vi "MapColor_array2Slide.vi"(6 "SlideValue\nIN":cluster{i32, i32, i32, i32, i32, i32, i32}(slide) scale=1.0..127.0, 7 "numSliders\n(optional)":i32=3, 8 "colormap":u32[](array[numeric])=[0, 196608, 393216, 589824, 786432, 983040, 1179648, 1376256, 1572864, 1769472, 1966080, 2162688, 2359296, 2555904, 2752512, 2949120, 3145728, 3342336, 3538944, 3735552, 3932160, 4128768, 4325376, 4521984, 4718592, 4915200, 5111808, 5308416, 5505024, 5701632, 5898240, 6094848, 6291456, 6488064, 6684672, 6881280, 7077888, 7274496, 7471104, 7667712, 7864320, 8060928, 8257536, 8454144, 8650752, 8847360, 9043968, 9240576, 9437184, 9633792, 9830400, 10027008, 10223616, 10420224, 10616832, 10813440, 11010048, 11206656, 11403264, 11599872, 11796480, 11993088, 12189696, 12386304, 12582912, 12779520, 12976128, 13172736, 13369344, 13565952, 13762560, 13959168, 14155776, 14352384, 14548992, 14745600, 14942208, 15138816, 15335424, 15532032, 15728640, 15925248, 16121856, 16318464, 16515072, 16711680, 16712448, 16713216, 16713984, 16714752, 16715520, 16716288, 16717056, 16717824, 16718592, 16719360, 16720128, 16720896, 16721664, 16722432, 16723200, 16723968, 16724736, 16725504, 16726272, 16727040, 16727808, 16728576, 16729344, 16730112, 16730880, 16731648, 16732416, 16733184, 16733952, 16734720, 16735488, 16736256, 16737024, 16737792, 16738560, 16739328, 16740096, 16740864, 16741632, 16742400, 16743168, 16743936, 16744704, 16745472, 16746240, 16747008, 16747776, 16748544, 16749312, 16750080, 16750848, 16751616, 16752384, 16753152, 16753920, 16754688, 16755456, 16756224, 16756992, 16757760, 16758528, 16759296, 16760064, 16760832, 16761600, 16762368, 16763136, 16763904, 16764672, 16765440, 16766208, 16766976, 16767744, 16768512, 16769280, 16770048, 16770816, 16771584, 16772352, 16773120, 16773888, 16774656, 16775424, 16776192, 16776960, 16776963, 16776966, 16776969, 16776972, 16776975, 16776977, 16776980, 16776983, 16776986, 16776989, 16776992, 16776995, 16776998, 16777001, 16777004, 16777007, 16777009, 16777012, 16777015, 16777018, 16777021, 16777024, 16777027, 16777030, 16777033, 16777036, 16777038, 16777041, 16777044, 16777047, 16777050, 16777053, 16777056, 16777059, 16777062, 16777065, 16777068, 16777070, 16777073, 16777076, 16777079, 16777082, 16777085, 16777088, 16777091, 16777094, 16777097, 16777100, 16777102, 16777105, 16777108, 16777111, 16777114, 16777117, 16777120, 16777123, 16777126, 16777129, 16777132, 16777134, 16777137, 16777140, 16777143, 16777146, 16777149, 16777152, 16777155, 16777158, 16777161, 16777163, 16777166, 16777169, 16777172, 16777175, 16777178, 16777181, 16777184, 16777187, 16777190, 16777193, 16777195, 16777198, 16777201, 16777204, 16777207]) -> (0 "SlideValue\nOUT":cluster{i32, i32, i32, i32, i32, i32, i32}(slide) scale=1.0..127.0, 1 "ActiveColors":i32[](array[numeric]), 2 "ColorFine":u32(colorbox)=16711680, 3 "ColorArray":u32[](array[colorbox]), 4 "ColorRamp":u32[](array[colorbox])=[180, 263349, 526518, 789687, 1052856, 1316026, 1579195, 1842364, 2105533, 2368702, 2631871, 2895040, 3158209, 3421378, 3684548, 3947717, 4145094, 4408263, 4671432, 4934601, 5197770, 5460939, 5724108, 5987278, 6250447, 6513616, 6776785, 7039954, 7303123, 7566292, 7829461, 8092630, 8355800, 8618969, 8882138, 9145307, 9408476, 9671645, 9934814, 10197983, 10461152, 10724322, 10987491, 11250660, 11513829, 11776998, 12040167, 12303336, 12500713, 12763882, 13027052, 13290221, 13553390, 13816559, 14079728, 14342897, 14606066, 14869235, 15132404, 15395574, 15658743, 15921912, 16185081, 16448250, 16448250, 16447222, 16446194, 16445166, 16444138, 16443110, 16442082, 16506590, 16505562, 16504534, 16503506, 16502478, 16501450, 16500422, 16499394, 16498366, 16497595, 16496567, 16495539, 16560047, 16559019, 16557991, 16556963, 16555935, 16554907, 16553879, 16552851, 16551823, 16550795, 16549767, 16548739, 16547711, 16612219, 16611191, 16610163, 16609135, 16608107, 16607079, 16606051, 16605023, 16603995, 16602967, 16601939, 16600911, 16599883, 16664391, 16663363, 16662335, 16661564, 16660536, 16659508, 16658480, 16657452, 16656424, 16655396, 16654368, 16653340, 16717848, 16716820, 16715792, 16714764, 16713736, 16712708, 16711680] caption="Color Ramp", 5 "ColorInizio":u32(colorbox)=180)   [LabVIEW 2010]
panel:
  out "array":i32[](array[numeric])
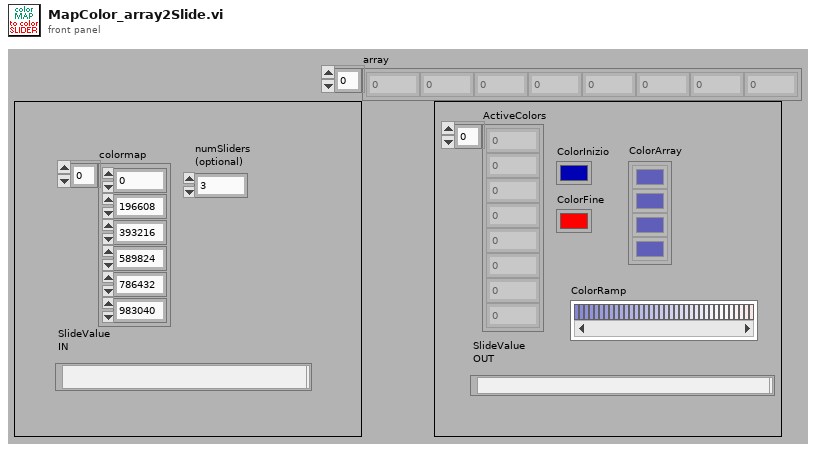
[diagram p1: front panel]
types:
  T1 = cluster{"SlideValue\nIN[0]":i32, "SlideValue\nIN[1]":i32, "SlideValue\nIN[2]":i32, "SlideValue\nIN[3]":i32, "SlideValue\nIN[4]":i32, "SlideValue\nIN[5]":i32, "SlideValue\nIN[6]":i32}
  T2 = cluster{"[0]":i32, "[1]":i32, "[2]":i32, "[3]":i32, "[4]":i32, "[5]":i32, "[6]":i32}
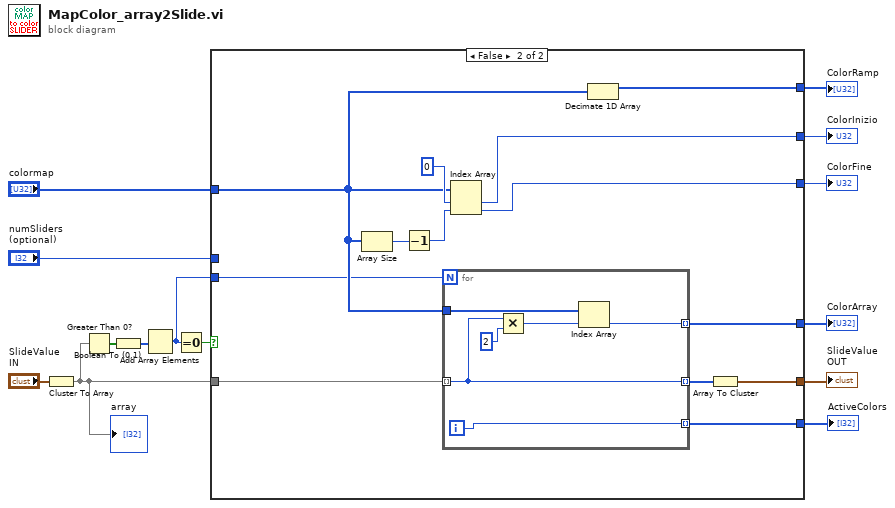
[diagram p0: block diagram]
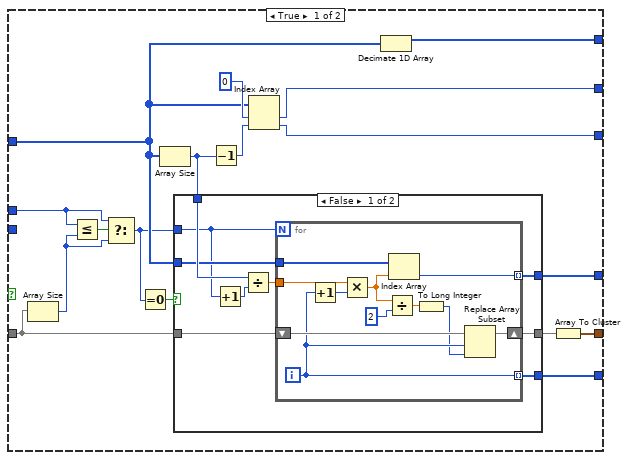
[diagram p2: hidden frame]
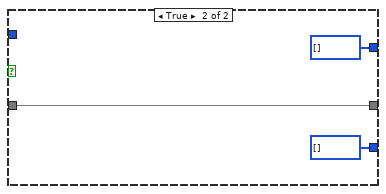
[diagram p3: hidden frame]
diagram:
  n1 = Cluster To Array(cluster="SlideValue\nIN") -> (array=w5:i32[])
  "array" <- w5
  n2 = Greater Than 0?(x=w5) -> (x > 0?=w4:bool[])
  n3 = Boolean To (0,1)(Boolean=w4) -> (0, 1=w3:i16[])
  n4 = Add Array Elements(numeric array=w3) -> (sum=w1:i16)
  n5 = Equal To 0?(x=w1) -> (x = 0?=w2:bool)
  n6 = case shown="False" w2 {
    tunnel: "numSliders\n(optional)" -> [w26 _]
    tunnel: [w25 w64] -> w12
    tunnel: [w24 w63] -> w11
    tunnel: [w23 w57] -> w10
    tunnel: [w21 w62] -> w9
    tunnel: [w20 w61] -> w8
    tunnel: [w19 w60] -> w7
    tunnel: w5 -> [w18 w58]
    tunnel: "colormap" -> [w17 w59]
    tunnel: w1 -> [_ w56]
    frame True {
      n7 = Array Size(array=w18) -> (size(s)=w22:i32)
      n8 = Less Or Equal?(x=w26, y=w22) -> (x <= y?=w27:bool)
      n9 = Select(t=w26, s=w27, f=w22) -> (s? t:f=w16:i32)
      n10 = Equal To 0?(x=w16) -> (x = 0?=w15:bool)
      n11 = Array Size(array=w17) -> (size(s)=w29:i32)
      n12 = case shown="False" w15 {
        tunnel: w29 -> [w40 _]
        tunnel: [w37 w54] -> w28
        tunnel: [w36 u32[] []] -> w24
        tunnel: [w35 i32[] []] -> w21
        tunnel: w18 -> [w34 w54]
        tunnel: w17 -> [w33 _]
        tunnel: w16 -> [w32 _]
        frame False {
          n13 = Increment(x=w32) -> (x+1=w38:i32)
          n14 = Divide(x=w40, y=w38) -> (x/y=w39:dbl)
          n15 = for {
            N: w32 -> [_]
            tunnel: w33 -> [w51]
            tunnel: w39 -> [w50]
            tunnel: [w49] -> w36 mode=indexing
            tunnel: [w42] -> w35 mode=indexing
            shift-right: [w43] -> w37
            shift-left: w34 -> [w45]
            i -> [w42]
            n16 = Increment(x=w42) -> (x+1=w48:i32)
            n17 = Multiply(x=w50, y=w48) -> (x*y=w46:dbl)
            n18 = Divide(x=w46, y=2) -> (x/y=w44:dbl)
            n19 = Index Array(array=w51, index=w46) -> (element=w49:u32)
            n20 = To Long Integer(number=w44) -> (32bit integer=w41:i32)
            n21 = Replace Array Subset(array=w45, new element=w41, index=w42) -> (w43:i32[])
          }
        }
        frame True {
        }
      }
      n22 = Decrement(x=w29) -> (x-1=w30:i32)
      n23 = Index Array(array=w17, index #1=0 ("index"), index #2=w30) -> (element #1=w19:u32, element #2=w20:u32)
      n24 = Decimate 1D Array(w17) -> (w25:u32[])  [unwired: 1 out]
      n25 = Array To Cluster(array=w28) -> (cluster=w23:T1)
    }
    frame False {
      n26 = Array Size(array=w59) -> (size(s)=w65:i32)
      n27 = Decrement(x=w65) -> (x-1=w66:i32)
      n28 = for {
        N: w56 -> [_]
        tunnel: w59 -> [w73]
        tunnel: [w72] -> w63 mode=indexing
        tunnel: [w71] -> w62 mode=indexing
        tunnel: w58 -> [w68] mode=indexing
        tunnel: [w68] -> w55 mode=indexing
        i -> [w71]
        n29 = Multiply(x=w68, y=2) -> (x*y=w70:i32)
        n30 = Index Array(array=w73, index=w70) -> (element=w72:u32)
      }
      n31 = Index Array(array=w59, index #1=0 ("index"), index #2=w66) -> (element #1=w60:u32, element #2=w61:u32)
      n32 = Decimate 1D Array(w59) -> (w64:u32[])  [unwired: 1 out]
      n33 = Array To Cluster(array=w55) -> (cluster=w57:T2)
    }
  }
  "ColorInizio" <- w7
  "ColorFine" <- w8
  "ColorRamp" <- w12
  "ColorArray" <- w11
  "SlideValue\nOUT" <- w10
  "ActiveColors" <- w9
